vi "8-Greater than 10 on string.vi"() -> ()   [LabVIEW 2019]
panel:
  out "String":string
  out "Array":dbl[](array[numeric])
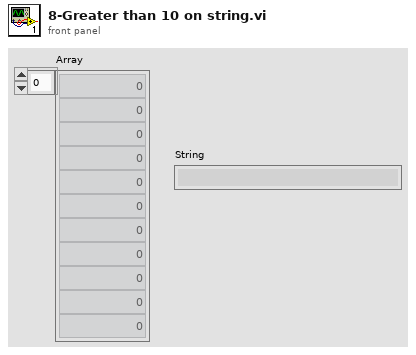
[diagram p1: front panel]
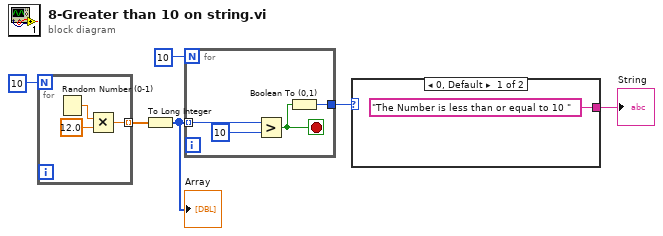
[diagram p0: block diagram]
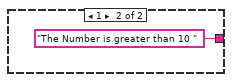
[diagram p2: hidden frame]
diagram:
  n1 = for {
    N: 10 -> [_]
    tunnel: [w7] -> w5 mode=indexing
    n2 = Random Number (0-1)() -> (number: 0 to 1=w9:dbl)
    n3 = Multiply(x=w9, y=12.0 ("x*y")) -> (x*y=w7:dbl)
  }
  n4 = To Long Integer(number=w5) -> (32bit integer=w3:i32[])
  "Array" <- w3
  n5 = for {
    N: 10 -> [_]
    tunnel: w3 -> [w13] mode=indexing
    tunnel: [w10] -> w1
    stop <- w11 stop-if-true
    n6 = Greater?(x=w13, y=10) -> (0:w11:bool)
    n7 = Boolean To (0,1)(Boolean=w11) -> (0, 1=w10:i16)
  }
  n8 = case shown="0, Default" w1 {
    tunnel: ["The Number is less than or equal to 10 " "The Number is greater than 10 "] -> w2
    frame 0, Default {
    }
    frame 1 {
    }
  }
  "String" <- w2
